vi "Read Strict refs box.vi"(8 "error in (no error)":errorcluster, 11 "BLE context in":refnum<class "BLE context.lvclass">) -> (0 "error out":errorcluster, 2 "Strict refs box":T1, 3 "BLE context out":refnum<class "BLE context.lvclass">)   [LabVIEW 2015, in "BLE context.lvclass"]
uses:
  BLE context.lvclass
  ctrls/RefsBox.ctl
  BLE context.lvclass/BLE context.ctl
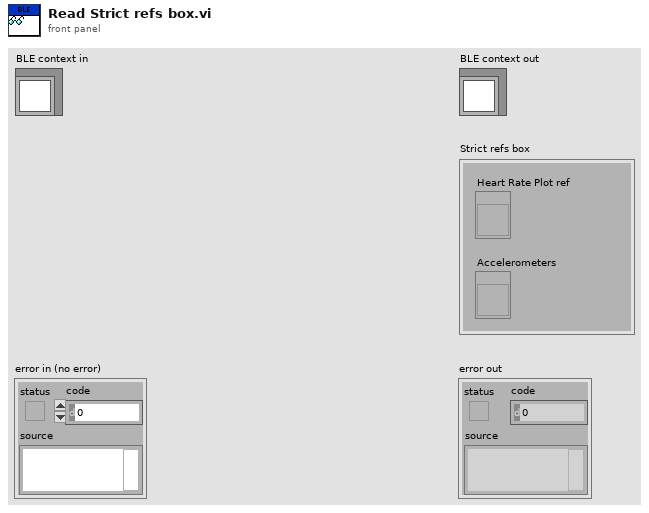
[diagram p1: front panel]
types:
  T1 = typedef "RefsBox.ctl" = cluster{"Heart Rate Plot ref":refnum<vi>, "Accelerometers":refnum<vi>}
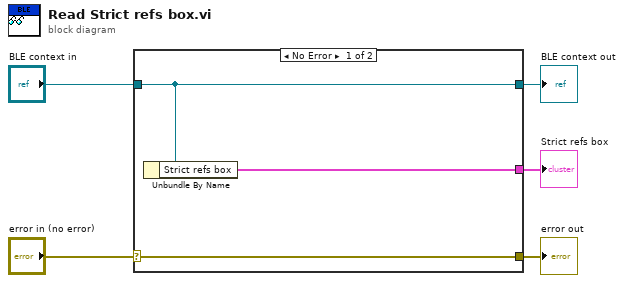
[diagram p0: block diagram]
diagram:
  n1 = case shown="No Error" "error in (no error)" {
    selector: "error in (no error)" -> [w8 w9]
    tunnel: [w8 w9] -> w4
    tunnel: [w7 w10] -> w2
    tunnel: "BLE context in" -> [w7 w10]
    tunnel: [w6 _] -> w1
    frame No Error {
      n2 = Unbundle By Name(w7) -> ("Strict refs box"=w6:T1)
    }
    frame Error {
    }
  }
  "error out" <- w4
  "BLE context out" <- w2
  "Strict refs box" <- w1
